vi "Test Deserialize Arrays.vi"(8 "error in (no error)":errorcluster) -> (0 "error out":errorcluster)   [LabVIEW 2013]
uses:
  src/Serializer/JSON Serializer/JSON Serializer.lvclass
  src/Deserializer/JSON Deserializer/JSON Deserializer.lvclass
  <vilib>/addons/_JKI Toolkits/Caraya/classes/Test/Test.lvclass
  <vilib>/addons/_JKI Toolkits/Caraya/classes/Assert/Assert.lvclass
  src/JKI JSON Serialization.lvlib
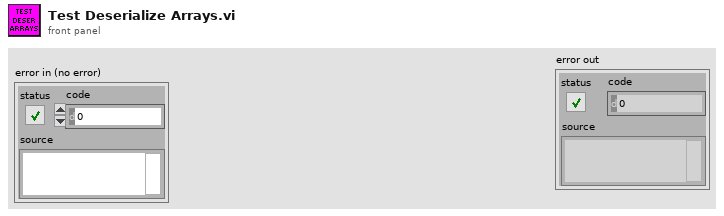
[diagram p1: front panel]
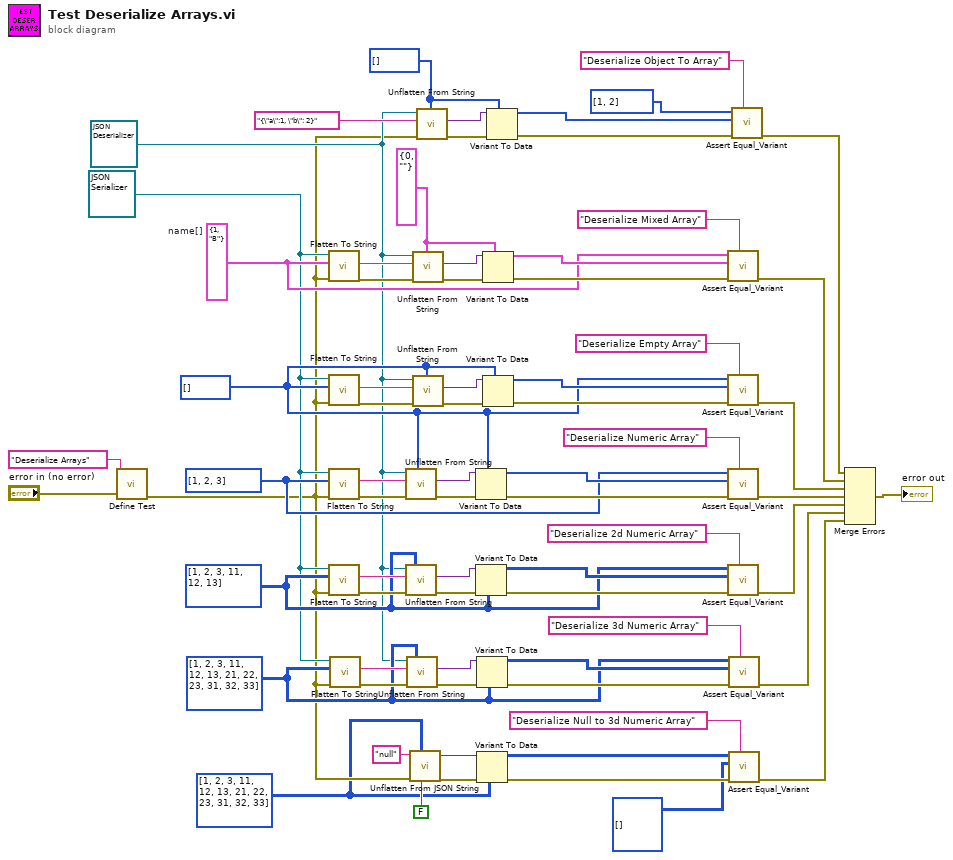
[diagram p0: block diagram]
diagram:
  w1 = i32[][][] [[[1, 2, 3], [11, 12, 13]], [[21, 22, 23], [31, 32, 33]]]
  w15 = i32[][][] [[[1, 2, 3], [11, 12, 13]], [[21, 22, 23], [31, 32, 33]]]
  w23 = i32[][] [[1, 2, 3], [11, 12, 13]]
  w34 = i32[] []
  w42 = i32[] [1, 2, 3]
  w41 = i32[] []
  w57 = cluster{"a":i32, "b":string} {"a"=0, "b"=""} ("name[]")
  w58 = cluster{"a":i32, "b":string} {"a"=1, "b"="B"}  # name[]
  w9 = refnum<class "JSON Deserializer.lvclass"> refnum ("Deserializer in")
  w10 = refnum<class "JSON Serializer.lvclass"> refnum ("JKI JSON Serialization.lvlib:JSON Serializer.lvclass")
  n1 = call <vilib>:"Define Test.vi"("error in (no error)"="error in (no error)", "Label (VI Title)"="Deserialize Arrays") -> ("error out"=w4:errorcluster)  [unwired: 9 in]
  n2 = call-dynamic "Flatten To String.vi"("error in (no error)"=w4, "Variant"=w58, "JSON Serializer in"=w10) -> ("error out"=w65:errorcluster, "String"=w64:string)  [unwired: 6 in, 1 out]
  n3 = call-dynamic "Flatten To String.vi"("error in (no error)"=w4, "Variant"=w41, "JSON Serializer in"=w10) -> ("error out"=w54:errorcluster, "String"=w53:string)  [unwired: 6 in, 1 out]
  n4 = call-dynamic "Flatten To String.vi"("error in (no error)"=w4, "Variant"=w42, "JSON Serializer in"=w10) -> ("error out"=w46:errorcluster, "String"=w45:string)  [unwired: 6 in, 1 out]
  n5 = call-dynamic "Flatten To String.vi"("error in (no error)"=w4, "Variant"=w23, "JSON Serializer in"=w10) -> ("error out"=w28:errorcluster, "String"=w27:string)  [unwired: 6 in, 1 out]
  n6 = call-dynamic "Flatten To String.vi"("error in (no error)"=w4, "Variant"=w15, "JSON Serializer in"=w10) -> ("error out"=w19:errorcluster, "String"=w18:string)  [unwired: 6 in, 1 out]
  n7 = call-dynamic "Unflatten From String.vi"("Type and Defaults"=w41, "error in (no error)"=w46, "String"=w45, "Deserializer in"=w9) -> ("error out"=w48:errorcluster, "Variant"=w47:variant)  [unwired: 5 in, 1 out]
  n8 = call-dynamic "Unflatten From String.vi"("Type and Defaults"=w23, "error in (no error)"=w28, "String"=w27, "Deserializer in"=w9) -> ("error out"=w30:errorcluster, "Variant"=w29:variant)  [unwired: 5 in, 1 out]
  n9 = call-dynamic "Unflatten From String.vi"("Type and Defaults"=w15, "error in (no error)"=w19, "String"=w18, "Deserializer in"=w9) -> ("error out"=w21:errorcluster, "Variant"=w20:variant)  [unwired: 5 in, 1 out]
  n10 = call "Unflatten From JSON String.vi"("Nulls as Defaults (T)"=FALSE, "Type and Defaults"=w1, "error in (no error)"=w4, "JSON String"="null") -> ("error out"=w7:errorcluster, "Variant"=w8:variant)  [unwired: 6 in]
  n11 = call-dynamic "Unflatten From String.vi"("Type and Defaults"=w57, "error in (no error)"=w65, "String"=w64, "Deserializer in"=w9) -> ("error out"=w63:errorcluster, "Variant"=w62:variant)  [unwired: 5 in, 1 out]
  n12 = call-dynamic "Unflatten From String.vi"("Type and Defaults"=w41, "error in (no error)"=w54, "String"=w53, "Deserializer in"=w9) -> ("error out"=w52:errorcluster, "Variant"=w51:variant)  [unwired: 5 in, 1 out]
  n13 = call-dynamic "Unflatten From String.vi"("Type and Defaults"=w34, "error in (no error)"=w4, "String"="{\"a\":1, \"b\": 2}", "Deserializer in"=w9) -> ("error out"=w39:errorcluster, "Variant"=w38:variant)  [unwired: 5 in, 1 out]
  n14 = Variant To Data(error in=w48, type=w41, Variant=w47) -> (data=w43:i32[], error out=w44:errorcluster)
  n15 = Variant To Data(error in=w30, type=w23, Variant=w29) -> (data=w25:i32[][], error out=w26:errorcluster)
  n16 = Variant To Data(error in=w21, type=w15, Variant=w20) -> (data=w16:i32[][][], error out=w17:errorcluster)
  n17 = Variant To Data(error in=w7, type=w1, Variant=w8) -> (data=w3:i32[][][], error out=w12:errorcluster)
  n18 = Variant To Data(error in=w63, type=w57, Variant=w62) -> (data=w61:cluster{"a":i32, "b":string}, error out=w60:errorcluster)
  n19 = Variant To Data(error in=w52, type=w41, Variant=w51) -> (data=w50:i32[], error out=w49:errorcluster)
  n20 = Variant To Data(error in=w39, type=w34, Variant=w38) -> (data=w37:i32[], error out=w36:errorcluster)
  n21 = call <vilib>:"Assert Equal_Variant.vi"("Label"="Deserialize Mixed Array", "error in (no error)"=w60, "Y"=w61, "X"=w58) -> ("error out"=w59:errorcluster)  [unwired: 7 in]
  n22 = call <vilib>:"Assert Equal_Variant.vi"("Label"="Deserialize Empty Array", "error in (no error)"=w49, "Y"=w50, "X"=w41) -> ("error out"=w68:errorcluster)  [unwired: 7 in]
  n23 = call <vilib>:"Assert Equal_Variant.vi"("Label"="Deserialize Numeric Array", "error in (no error)"=w44, "Y"=w43, "X"=w42) -> ("error out"=w69:errorcluster)  [unwired: 7 in]
  n24 = call <vilib>:"Assert Equal_Variant.vi"("Label"="Deserialize 2d Numeric Array", "error in (no error)"=w26, "Y"=w25, "X"=w23) -> ("error out"=w24:errorcluster)  [unwired: 7 in]
  n25 = call <vilib>:"Assert Equal_Variant.vi"("Label"="Deserialize 3d Numeric Array", "error in (no error)"=w17, "Y"=w16, "X"=w15) -> ("error out"=w14:errorcluster)  [unwired: 7 in]
  n26 = call <vilib>:"Assert Equal_Variant.vi"("Label"="Deserialize Null to 3d Numeric Array", "error in (no error)"=w12, "Y"=i32[][][] [] ("data"), "X"=w3) -> ("error out"=w11:errorcluster)  [unwired: 7 in]
  n27 = call <vilib>:"Assert Equal_Variant.vi"("Label"="Deserialize Object To Array", "error in (no error)"=w36, "Y"=w37, "X"=i32[] [1, 2]) -> ("error out"=w35:errorcluster)  [unwired: 7 in]
  n28 = Merge Errors(w35, w59, w68, w69, w24, w14, w11) -> (→"error out":errorcluster)
